vi "Begin.vi"(11 "Image Size":T6=enum."160x120") -> (0 "error out":errorcluster)   [LabVIEW 2014]
doc: "Called before other user functions, this VI is expected to open initial I/O refnums, load in file data, and do all program initialization. Notice that the <B>error out</B> terminal is simply used for data flow. Wiring it to other structures or subVIs ensures that this VI runs first."
uses:
  <vilib>/Rock Robotics/WPI/Camera/WPI_CameraImageSize.ctl
  <vilib>/Rock Robotics/SystemInterfaces/DIO/FPGA_DIOChannel.ctl
  <vilib>/Rock Robotics/SystemInterfaces/DIO/FPGA_DIORelayChannel.ctl
  <vilib>/Rock Robotics/SystemInterfaces/DIO/FPGA_DIOPWMChannel.ctl
  <vilib>/Rock Robotics/WPI/Solenoid/WPI_SolenoidChannel.ctl
  <vilib>/Rock Robotics/WPI/Relay/WPI_RelayDirection.ctl
  <vilib>/Rock Robotics/WPI/Camera/WPI_CameraWhite Balance Values.ctl
  <vilib>/Rock Robotics/WPI/Camera/WPI_CameraExposure Values.ctl
  <vilib>/Rock Robotics/WPI/Camera/WPI_CameraFrameRate.ctl
  <vilib>/Rock Robotics/WPI/SafetyOutput/WPI_SafetyOutputConfigMenu.ctl
  <vilib>/Rock Robotics/WPI/DriverStation/WPI_DriverStationRobotMode2.ctl
  <vilib>/Rock Robotics/WPI/Joystick/WPI_JoystickDeviceEnum.ctl
  <vilib>/Rock Robotics/SystemInterfaces/Typedef/FPGA_TypedefDigitalModule.ctl
  <vilib>/Rock Robotics/SystemInterfaces/Typedef/FPGA_TypedefSolenoidModule.ctl
  <vilib>/Rock Robotics/WPI/RobotDrive/WPI_RobotDriveOpen2MotorWithJaguar.vi
  Robot Global Data.vi
  <vilib>/Rock Robotics/WPI/MotorControl/WPI_MotorControlOpen Talon.vi
  <vilib>/Rock Robotics/WPI/Solenoid/WPI_SolenoidOpenDouble.vi
  <vilib>/Rock Robotics/WPI/Compressor/WPI_CompressorGetSetRefNum.vi
panel:
  in  "Relay Direction 2":T1
  in  "Relay Channel":T2
  in  "Reverse Solenoid Channel 3":T3=enum."Solenoid 5"
  in  "Forward Solenoid Channel 3":T3=enum."Solenoid 6"
  in  "Forward Solenoid Channel 2":T3=enum."Solenoid 3"
  in  "Reverse Solenoid Channel 2":T3=enum."Solenoid 4"
  in  "Relay Direction":T1
  in  "Relay Channel Indexer":T2=enum."Relay 6"
  in  "PWM Channel Shooter 2":T4=enum."PWM 6"
  in  "Reverse Solenoid Channel":T3=enum."Solenoid 2"
  in  "Forward Solenoid Channel":T3
  in  "PWM Channel Shooter 1":T4=enum."PWM 7"
  in  "Relay Channel 2":T2=enum."Relay 2"
  in  "Pressure Switch DIO Channel":T5
  # "Encoders"
  # "Indexer"
  # "compressor"
  # "Shooter \nArm"
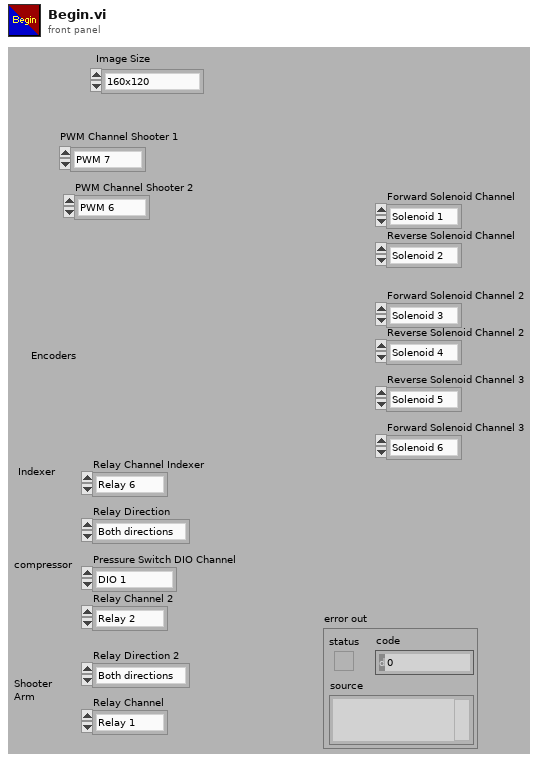
[diagram p1: front panel]
types:
  T1 = typedef "WPI_RelayDirection.ctl" = enum16{"Both directions", "Forward only", "Reverse only"}
  T2 = typedef "FPGA_DIORelayChannel.ctl" = enum8{"Relay 1", "Relay 2", "Relay 3", "Relay 4", "Relay 5", "Relay 6", "Relay 7", "Relay 8", "Invalid"}
  T3 = typedef "WPI_SolenoidChannel.ctl" = enum8{"Solenoid 1", "Solenoid 2", "Solenoid 3", "Solenoid 4", "Solenoid 5", "Solenoid 6", "Solenoid 7", "Solenoid 8", "Invalid"}
  T4 = typedef "FPGA_DIOPWMChannel.ctl" = enum8{"PWM 1", "PWM 2", "PWM 3", "PWM 4", "PWM 5", "PWM 6", "PWM 7", "PWM 8", "PWM 9", "PWM 10", "Invalid"}
  T5 = typedef "FPGA_DIOChannel.ctl" = enum8{"DIO 1", "DIO 2", "DIO 3", "DIO 4", "DIO 5", "DIO 6", "DIO 7", "DIO 8", "DIO 9", "DIO 10", "DIO 11", "DIO 12", "DIO 13", "DIO 14", "Invalid"}
  T6 = typedef "WPI_CameraImageSize.ctl" = enum16{"640x480", "320x240", "160x120"}
  T7 = typedef "FPGA_TypedefSolenoidModule.ctl" = enum16{"Solenoid Module 1", "Solenoid Module 2"}
  T8 = typedef "WPI_JoystickDeviceEnum.ctl" = enum16{"USB 0", "USB 1", "USB 2", "USB 3", "USB 4", "USB 5"}
  T9 = typedef "FPGA_TypedefDigitalModule.ctl" = enum16{"Digital Module 1", "Digital Module 2"}
  T10 = typedef "WPI_DriverStationRobotMode2.ctl" = enum16{"Autonomous Disabled", "Autonomous Enabled", "Teleop Disabled", "Teleop Enabled", "Disconnected", "Finish", "Test Disabled", "Test Enabled"}
  T11 = typedef "WPI_SafetyOutputConfigMenu.ctl" = enum16{"Enable", "Disable"}
  T12 = typedef "WPI_CameraFrameRate.ctl" = u32
  T13 = typedef "WPI_CameraExposure Values.ctl" = enum16{"Auto", "Flicker-free 50 Hz", "Flicker-free 60 Hz", "Hold current"}
  T14 = typedef "WPI_CameraWhite Balance Values.ctl" = enum16{"Auto", "Fixed indoor", "Fixed outdoor 1", "Fixed outdoor 2", "Fixed fluorescent 1", "Fixed fluorescent 2", "Hold current"}
  T15 = typedef "WPI_SolenoidDevRef.ctl" = cluster{"DevStatus":errorcluster, "Solenoid Module":T7, "Forward Solenoid Channel":T3, "Reverse Solenoid Channel":T3}
  T16 = typedef "WPI_JoystickDevRef.ctl" = cluster{"Device":T8}
  T17 = typedef "WPI_CameraDevRef.ctl" = cluster{"Camera Address":string, "CameraStatus":errorcluster, "Acquire Image Notifier":refnum<notifier>}
  T18 = typedef "WPI_RobotDriveDevRef.ctl" = cluster{"DevStatus":errorcluster, "Motors[]":T19[], "Square Inputs":bool, "Max Output":dbl}
  T19 = typedef "WPI_MotorControlDeviceRef.ctl" = cluster{"DeviceStatus":errorcluster, "Type":enum16{"PWM", "CAN"}, "PWM":cluster{"Digital Module":T9, "PWM Channel":T4, "DeadBand":T20}, "CAN":cluster{"Device Number":u8, "Control Mode":T21, "Semaphore":T22, "Max Vout":dbl}, "Invert":bool, "TransformRef":T23, "InvTransformRef":T23}
  T20 = typedef "WPI_PWMDeadband.ctl" = cluster{"Name":string, "maxPositivePwm":i32, "minPositivePwm":i32, "centerPwm":i32, "maxNegativePwm":i32, "minNegativePwm":i32, "angularRange":u16}
  T21 = typedef "WPI_CANJaguar_ControlMode.ctl" = enum8{"Percent VBus", "Current", "Speed", "Position", "Voltage"}
  T22 = typedef "Semaphore RefNum" = refnum<k1>
  T23 = typedef "WPI_PWMTransform_ConPane.ctl" = refnum<vi>
  T24 = typedef "WPI_RelayDevRef.ctl" = cluster{"DevStatus":errorcluster, "Relay Channel":T2, "Digital Module":T9, "Relay Direction":T1}
  T25 = typedef "WPI_CompressorDevRef.ctl" = cluster{"DevStatus":errorcluster, "DigitalInputDevRef":T26, "RelayDevRef":T24}
  T26 = typedef "WPI_DigitalInputDevRef.ctl" = cluster{"DevStatus":errorcluster, "DIO Channel":T5, "Digital Module":T9}
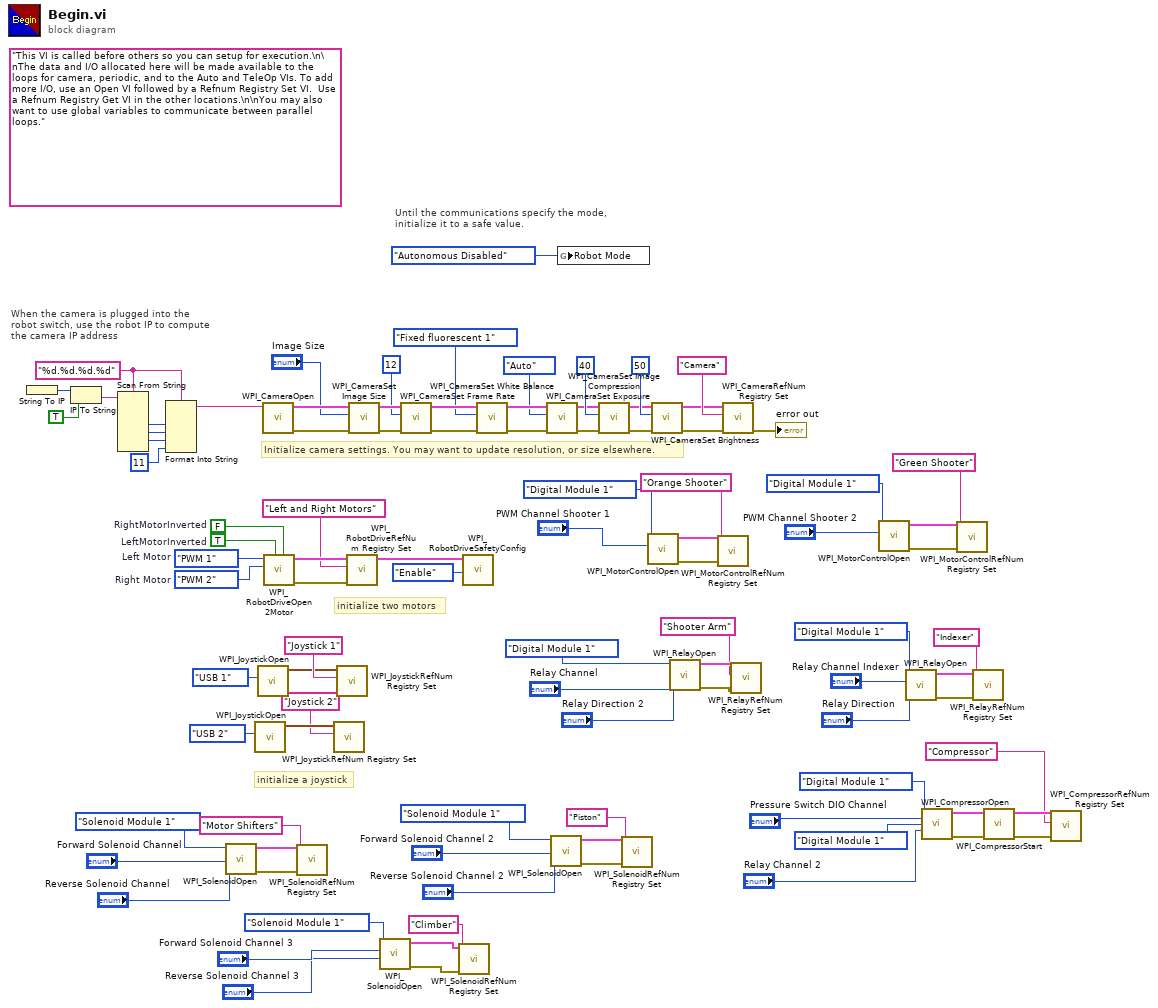
[diagram p0: block diagram]
diagram:
  w61 = "%d.%d.%d.%d" ("format string")
  (unwired) "This VI is called before others so you can setup for execution.\n\nThe data and I/O allocated here will be made available to the loops for camera, periodic, and to the Auto and TeleOp VIs. To add more I/O, use an Open VI followed by a Refnum Registry Set VI.  Use a Refnum Registry Get VI in the other locations.\n\nYou may also want to use global variables to communicate between parallel loops."
  w72 = FPGA_DIOPWMChannel."PWM 2"  # Right Motor
  w73 = FPGA_DIOPWMChannel."PWM 1"  # Left Motor
  w95 = TRUE  # LeftMotorInverted
  w96 = FALSE  # RightMotorInverted
  # "initialize a joystick"
  # "Until the communications specify the mode,\ninitialize it to a safe value."
  # "When the camera is plugged into the\nrobot switch, use the robot IP to compute\nthe camera IP address"
  # "initialize two motors"
  # "Initialize camera settings. You may want to update resolution, or size elsewhere."
  n1 = String To IP() -> (0:w68:u32)  [unwired: 1 in]
  n2 = IP To String(1:TRUE ("dot notation? (F)"), 2:w68) -> (0:w66:string)
  n3 = Scan From String(format string=w61, input string=w66) -> (output 1=w65:i32, output 2=w64:i32, output 3=w63:i32)  [unwired: 7 in, 3 out]
  n4 = Format Into String(format string=w61, w65, w64, w63, 11 ("Compression")) -> (resulting string=w57:string)  [unwired: 2 in, 1 out]
  n5 = call-poly <vilib>:"WPI_SolenoidOpen.vi"("Reverse Solenoid Channel"="Reverse Solenoid Channel", "Forward Solenoid Channel"="Forward Solenoid Channel", "Solenoid Module (Module 1)"=FPGA_TypedefSolenoidModule."Solenoid Module 1") -> ("error out"=w46:errorcluster, "SolenoidDevRef"=w47:T15)  [unwired: 7 in]
  n6 = call <vilib>:"WPI_JoystickOpen.vi"("JoystickDevice"=WPI_JoystickDeviceEnum."USB 2") -> ("JoystickDevRef"=w8:T16)  [unwired: 10 in]
  n7 = call <vilib>:"WPI_JoystickOpen.vi"("JoystickDevice"=WPI_JoystickDeviceEnum."USB 1") -> ("JoystickDevRef"=w55:T16)  [unwired: 10 in]
  n8 = call <vilib>:"WPI_CameraOpen.vi"("Camera Address"=w57) -> ("error out"=w82:errorcluster, "CameraDevRef"=w83:T17)  [unwired: 1 in, 8 out]
  n9 = call-poly <vilib>:"WPI_RobotDriveOpen2Motor.vi"("Right Motor Inverted"=w96, "Left Motor Inverted"=w95, "Right Motor"=w72, "Left Motor"=w73) -> ("error out"=w91:errorcluster, "RobotDriveDevRef"=w93:T18)  [unwired: 1 in, 5 out]
  n10 = call <vilib>:"WPI_SolenoidRefNum Registry Set.vi"("error in (no error)"=w46, "refnum name"="Motor Shifters", "SolenoidDevRef"=w47) -> ()  [unwired: 7 in, 2 out]
  n11 = call <vilib>:"WPI_JoystickRefNum Registry Set.vi"("refnum name"="Joystick 2", "JoystickDevRef"=w8) -> ()  [unwired: 8 in, 2 out]
  n12 = call <vilib>:"WPI_JoystickRefNum Registry Set.vi"("refnum name"="Joystick 1", "JoystickDevRef"=w55) -> ()  [unwired: 8 in, 2 out]
  n13 = call <vilib>:"WPI_RobotDriveRefNum Registry Set.vi"("error in (no error)"=w91, "refnum name"="Left and Right Motors", "RobotDriveDevRef"=w93) -> ("RobotDriveDevRef"=w60:T18)  [unwired: 8 out]
  n14 = call <vilib>:"WPI_CameraSet Image Size.vi"("error in (no error)"=w82, "Image Size"="Image Size", "CameraDevRef"=w83) -> ("error out"=w81:errorcluster, "CameraDevRef Out"=w84:T17)  [unwired: 7 out]
  n15 = call-poly <vilib>:"WPI_SolenoidOpen.vi"("Reverse Solenoid Channel"="Reverse Solenoid Channel 3", "Forward Solenoid Channel"="Forward Solenoid Channel 3", "Solenoid Module (Module 1)"=FPGA_TypedefSolenoidModule."Solenoid Module 1") -> ("error out"=w5:errorcluster, "SolenoidDevRef"=w6:T15)  [unwired: 7 in]
  n16 = call <vilib>:"WPI_CameraSet Frame Rate.vi"("error in (no error)"=w81, "Frame Rate (fps)"=T12 12, "CameraDevRef"=w84) -> ("error out"=w80:errorcluster, "CameraDevRef Out"=w86:T17)  [unwired: 7 out]
  n17 = call <vilib>:"WPI_SolenoidRefNum Registry Set.vi"("error in (no error)"=w5, "refnum name"="Climber", "SolenoidDevRef"=w6) -> ()  [unwired: 7 in, 2 out]
  n18 = call <vilib>:"WPI_RobotDriveSafetyConfig.vi"("mode"=WPI_SafetyOutputConfigMenu."Enable", "RobotDriveDevRef"=w60) -> ()  [unwired: 8 in, 2 out]
  n19 = call <vilib>:"WPI_CameraSet White Balance.vi"("error in (no error)"=w80, "White Balance"=WPI_CameraWhite_Balance_Values."Fixed fluorescent 1", "CameraDevRef"=w86) -> ("error out"=w79:errorcluster, "CameraDevRef Out"=w85:T17)  [unwired: 7 out]
  n20 = call <vilib>:"WPI_CameraSet Exposure.vi"("error in (no error)"=w79, "Exposure"=WPI_CameraExposure_Values."Auto", "CameraDevRef"=w85) -> ("error out"=w78:errorcluster, "CameraDevRef Out"=w88:T17)  [unwired: 7 out]
  n21 = call-poly <vilib>:"WPI_SolenoidOpen.vi"("Reverse Solenoid Channel"="Reverse Solenoid Channel 2", "Forward Solenoid Channel"="Forward Solenoid Channel 2", "Solenoid Module (Module 1)"=FPGA_TypedefSolenoidModule."Solenoid Module 1") -> ("error out"=w11:errorcluster, "SolenoidDevRef"=w10:T15)  [unwired: 7 in]
  n22 = global write "Robot Global Data.vi" "Robot Mode"(WPI_DriverStationRobotMode2."Autonomous Disabled" ("Robot Mode")) -> ()
  n23 = call <vilib>:"WPI_CameraSet Image Compression.vi"("error in (no error)"=w78, "Compression"=40, "CameraDevRef"=w88) -> ("error out"=w77:errorcluster, "CameraDevRef Out"=w87:T17)  [unwired: 7 out]
  n24 = call <vilib>:"WPI_SolenoidRefNum Registry Set.vi"("error in (no error)"=w11, "refnum name"="Piston", "SolenoidDevRef"=w10) -> ()  [unwired: 7 in, 2 out]
  n25 = call-poly <vilib>:"WPI_MotorControlOpen.vi"("PWM Channel"="PWM Channel Shooter 1", "Digital Module (Module 1)"=FPGA_TypedefDigitalModule."Digital Module 1") -> ("error out"=w49:errorcluster, "MotorControlDeviceRef"=w50:T19)  [unwired: 8 in]
  n26 = call <vilib>:"WPI_CameraSet Brightness.vi"("error in (no error)"=w77, "Brightness"=50, "CameraDevRef"=w87) -> ("error out"=w75:errorcluster, "CameraDevRef Out"=w76:T17)  [unwired: 7 out]
  n27 = call <vilib>:"WPI_RelayOpen.vi"("Relay Direction"="Relay Direction 2", "Relay Channel"="Relay Channel", "Digital Module (Module 1)"=FPGA_TypedefDigitalModule."Digital Module 1") -> ("error out"=w18:errorcluster, "RelayDevRef"=w17:T24)  [unwired: 7 in]
  n28 = call <vilib>:"WPI_MotorControlRefNum Registry Set.vi"("error in (no error)"=w49, "refnum name"="Orange Shooter", "MotorControlDevRef"=w50) -> ()  [unwired: 7 in, 2 out]
  n29 = call <vilib>:"WPI_CameraRefNum Registry Set.vi"("error in (no error)"=w75, "refnum name"="Camera", "CameraDevRef"=w76) -> ("error out"=→"error out":errorcluster)  [unwired: 8 out]
  n30 = call <vilib>:"WPI_RelayRefNum Registry Set.vi"("error in (no error)"=w18, "refnum name"="Shooter Arm", "RelayDevRef"=w17) -> ()  [unwired: 7 in, 2 out]
  n31 = call-poly <vilib>:"WPI_MotorControlOpen.vi"("PWM Channel"="PWM Channel Shooter 2", "Digital Module (Module 1)"=FPGA_TypedefDigitalModule."Digital Module 1") -> ("error out"=w29:errorcluster, "MotorControlDeviceRef"=w31:T19)  [unwired: 8 in]
  n32 = call <vilib>:"WPI_RelayOpen.vi"("Relay Direction"="Relay Direction", "Relay Channel"="Relay Channel Indexer", "Digital Module (Module 1)"=FPGA_TypedefDigitalModule."Digital Module 1") -> ("error out"=w23:errorcluster, "RelayDevRef"=w27:T24)  [unwired: 7 in]
  n33 = call <vilib>:"WPI_CompressorOpen.vi"("Pressure Switch Digital Module (Module 1)"=FPGA_TypedefDigitalModule."Digital Module 1", "Pressure Switch DIO Channel"="Pressure Switch DIO Channel", "Relay Digital Module (Module 1)"=FPGA_TypedefDigitalModule."Digital Module 1", "Relay Channel"="Relay Channel 2") -> ("CompressorDevRef"=w37:T25, "error out"=w36:errorcluster)  [unwired: 10 in]
  n34 = call <vilib>:"WPI_MotorControlRefNum Registry Set.vi"("error in (no error)"=w29, "refnum name"="Green Shooter", "MotorControlDevRef"=w31) -> ()  [unwired: 7 in, 2 out]
  n35 = call <vilib>:"WPI_RelayRefNum Registry Set.vi"("error in (no error)"=w23, "refnum name"="Indexer", "RelayDevRef"=w27) -> ()  [unwired: 7 in, 2 out]
  n36 = call <vilib>:"WPI_CompressorStart.vi"("error in (no error)"=w36, "CompressorDevRef"=w37) -> ("error out"=w34:errorcluster, "CompressorDevRef"=w35:T25)  [unwired: 8 in]
  n37 = call <vilib>:"WPI_CompressorRefNum Registry Set.vi"("error in (no error)"=w34, "refnum name"="Compressor", "CompressorDevRef"=w35) -> ()  [unwired: 7 in, 2 out]
